vi "GUI main.vi"() -> ()   [LabVIEW 2020]
doc: "GUI of the control sotware. Entry VI that runs the whole control sotware."
uses:
  General DC meter/Type definitions/DC meter.ctl
  General DC meter/Type definitions/DC meter type.ctl
  General AC source/Type definitions/AC Source.ctl
  General AC source/Type definitions/AC Source type.ctl
  CE Measurement/Type definitions/CE measurement.ctl
  Utilities/Type definitions/Common properties.ctl
  FR Measurement/Type definitions/FR measuement.ctl
  General PJVS driver/Type definitions/PJVS.ctl
  General PJVS driver/Type definitions/PJVS Type.ctl
  external libraries/acsvcontrol-driver/Public/Type Definitions/Timeouts.ctl
  external libraries/JV modified NPL Bias source/DataSocketCluster external.ctl
  SS Measurement/Type definitions/SS measurement.ctl
  DG Measurement/DG measurement.ctl
  72cf5302-2c4c-4f5f-a6af-2a69e50c2212.vi
  <vilib>/Utility/error.llb/Error Cluster From Error Code.vi
  <vilib>/ErrorRing/Error Ring.xnode
  external libraries/varilib/varilib.lvlib
  external libraries/acsvcontrol-driver/ACSVcontrol-driver.lvlib
panel:
  out "DG measurement":T1={"Sampling frequencies (Hz)"=[10000000.0], "Requested PJVS frequencies (Hz)"=[1000.0], "Requested PJVS waveform amplitudes (V)"=[0.707], "Record lengths (multiples of PJVS periods)"=[10000.0], "Requested PJVS steps"=[20], "Switch position"=0.0, "Settle down after PJVS change (s)"=1.0, "Rs"=0, "Re"=0, "Algorithm"="TWM-PJVSSubS", "Calculate results"=FALSE, "Data folder"=path "", "TWM data directories"=[], "TWM data directories relative"=[], "DG measurement info files"=[], "Set PJVS frequencies (Hz)"=[1000.0], "Set PJVS reference voltages array of vector cluster"=[], "Set PJVS steps"=[1000]} {"Set PJVS frequencies (Hz)" format="%#_3p"; "Set PJVS reference voltages array of vector cluster"."PJVS reference voltages vector" format="%#_3p"; "Requested PJVS frequencies (Hz)" format="%#_3p"; "Record lengths (multiples of PJVS periods)" format="%#_3p"; "Sampling frequencies (Hz)" format="%#_3p"; "Requested PJVS waveform amplitudes (V)" format="%#_3p"}
  in  "DG setup":bool
  in  "DG measure":bool
  out "AC sync source":T2
  in  "DC manual":bool
  out "SS measurement":T4={"Signal frequencies (Hz)"=[1000.0], "Signal amplitudes (V)"=[0.707], "Sampling frequencies (Hz)"=[10000000.0], "Record lengths (multiples of periods)"=[10000.0], "Calculate results"=FALSE, "Algorithm"="TWM-WFFT", "TWM data directories"=[], "TWM data directories relative"=[], "Settle down after AC source change (s)"=1.0, "PJVS frequencies (Hz)"=[1000.0], "PJVS reference voltages array of vector cluster"=[{"PJVS reference voltages vector"=[]}], "Requested PJVS steps"=[20], "Measure CE"=FALSE, "Measure CE before"=FALSE, "Measure CE after"=FALSE, "Single point CE measurement"=FALSE, "original CE template path"=path "", "new CE template path before SS"=path "", "new CE template path before SS relative"=path "", "new CE template path after SS"=path "", "new CE template path after SS relative"=path "", "original CE fit path"=path "", "new CE fit path before SS"=path "", "new CE fit path before SS relative"=path "", "new CE fit path after SS"=path "", "new CE fit path after SS relative"=path "", "Measure digitizer gain"=FALSE, "Measure digitizer gain before"=FALSE, "Measure digitizer gain after"=FALSE, "Digitizer gain"=0.0, "Data folder"=path "", "FR fit path"=path "", "new FR fit path relative"=path "", "Rs"=0, "Re"=0, "SS measurement info files"=[]} {"PJVS reference voltages array of vector cluster"."PJVS reference voltages vector" format="%#_3p"; "PJVS frequencies (Hz)" format="%#_3p"; "Record lengths (multiples of periods)" format="%#_3p"; "Sampling frequencies (Hz)" format="%#_3p"; "Signal amplitudes (V)" format="%#_3p"; "Signal frequencies (Hz)" format="%#_3p"}
  out "PJVS":T5={"PJVS type"=enum."AC-supraVOLTcontrol", "Status Refnum"=refnum, "AC-supraVOLTcontrol"={"IP address:port (0.0.0.0:0000)"="0.0.0.0:0000", "Timeouts"={"TCP Read & Write (ms)"=7000, "Sensors readout"=5000, "PJVS setup"=10000, "Nullmeter readout"=5000, "Multiplexer setup"=3000, "57XX setup"=15000, "Generator setup"=5000, "Synthesizer setup"=3000, "Sampler readout"=10000}, "Simulation mode"=FALSE, "Debug mode"=FALSE}, "NPL bias source"={"DataSocketCluster"={"Server Machine"="CZC105BD8M", "Client Machine"="localhost", "Data"="P2", "TimeStamp"=0.0, "Count"=1, "Target Process"="General Server"}}, "Manual PJVS"={"PJVS frequency (Hz)"=0.0, "Reference voltages (V)"=[], "File with PJVS voltages"=path ""}, "VTT PJVS"={"some VTT only property"=""}} {"NPL bias source"."DataSocketCluster"."TimeStamp" format="%.2f"}
  out "FR measurement":T9={"Measurement frequencies (Hz)"=[1000.0, 10000.0, 1000.0], "Sampling frequency (Hz)"=500000.0, "Signal amplitude (V)"=4.5, "AC-DC settle time (s)"=20.0, "Record length (multiples of period)"=[1000.0, 10000.0, 1000.0], "Measurement template file"=path "", "Row of START keyword"=0, "Row of STOP keyword"=0, "Calculate RMS from samples"=FALSE, "AC-DC warm up time (s)"=300.0, "Measurement template line"=[], "DC meter readings No."=10, "Algorithm"="TWM-WFFT", "Simultaneous measurement"=FALSE, "Recalculate-skip already calculated"=FALSE} {"Record length (multiples of period)" format="%#_3p"; "Sampling frequency (Hz)" format="%#_3p"; "Measurement frequencies (Hz)" format="%#_3p"}
  in  "DS setup":bool
  in  "DS measure":bool
  in  "SS setup":bool
  in  "SS measure":bool
  out "Common properties":T10={"Measurement status ref"=refnum, "TWM Status ref"=refnum, "Abort ref"=refnum, "Skip waiting ref"=refnum, "GNU Octave path"=path "C:/Program Files/GNU Octave/Octave-6.2.0/mingw64/bin", "TWM+QWTB path"=path "C:/Users/labina/Desktop/TWM-1.8.7.0-full/octprog", "lvlib path"=path "D:/martin/WAC/WACsw - github/control_software/Filter function meter/external libraries/GOLPI 0.7.3.1 source distribution LV 20.0 32 bit/lv_proc.dll", "TWM pipe"="\\\\.\\pipe\\TWM:server", "PJVS status ref"=refnum, "WAC path"=path ""}
  out "CE measurement":T11={"Signal frequencies (Hz) T"=[1000.0], "Signal amplitudes (V) T"=[0.707], "Sampling frequencies (Hz) T"=[10000000.0], "Record lengths (multiples of periods) T"=[10000.0], "TWM data root directory"=path "", "TWM mreasurements directories"=[], "Calculate RMS from samples"=FALSE, "Algorithm to use"="TWM-WFFT", "Quantity to read"="TWM-WFFT", "Settle down after AC source change (s) T"=1.0, "Skip PJVS setup"=FALSE, "Measurement template file"=path "", "Row of START keyword T"=0, "Row of STOP keyword T"=0, "Measurement template line T"=[], "Switch position T"=[10000.0], "FR fit mat file T"=path "", "Recalculate-skip already calculated"=FALSE} {"Switch position T" format="%#_3p"; "Record lengths (multiples of periods) T" format="%#_3p"; "Sampling frequencies (Hz) T" format="%#_3p"; "Signal amplitudes (V) T" format="%#_3p"; "Signal frequencies (Hz) T" format="%#_3p"}
  in  "CE setup":bool
  in  "CE measure":bool
  out "AC Source":T2
  out "DC meter":T12={"DC meter type"=enum."H/A/K 3458", "DC meter VISA"="", "NPLC"=10.0, "status ref"=refnum}
  in  "PJVS setup":bool
  out "PJVS status":string caption="PJVS:"
  out "gui_to_hide":refnum<vi>[](array[refnum])
  in  "Skip waiting":bool caption="Abort"
  in  "DCV setup":bool
  out "DC meter status":string caption="DC meter:"
  out "Measurement status:":string
  in  "AC setup":bool
  in  "FR measure":bool
  out "gui_unlock_for_measure":refnum<vi>[](array[refnum])
  out "gui_to_lock":refnum<vi>[](array[refnum])
  in  "FR setup":bool
  in  "Abort":bool
  out "AC source status":string caption="AC source:"
  out "TWM status":string caption="TWM:"
  in  "TWM setup":bool
  in  "About":bool
  in  "Quit":bool
  in  "ACmanual":bool
  in  "PJVSmanual":bool
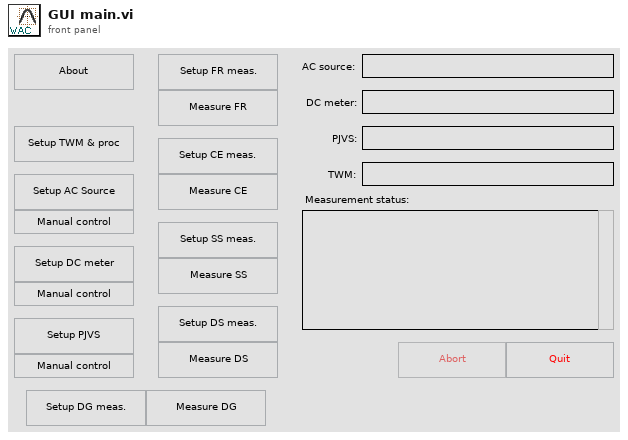
[diagram p1: front panel]
types:
  T1 = typedef "DG measurement.ctl" = cluster{"Sampling frequencies (Hz)":dbl[], "Requested PJVS frequencies (Hz)":dbl[], "Requested PJVS waveform amplitudes (V)":dbl[], "Record lengths (multiples of PJVS periods)":dbl[], "Requested PJVS steps":u32[], "Switch position":dbl, "Settle down after PJVS change (s)":dbl, "Rs":i32, "Re":i32, "Algorithm":string, "Calculate results":bool, "Data folder":path, "TWM data directories":path[], "TWM data directories relative":path[], "DG measurement info files":path[], "Set PJVS frequencies (Hz)":dbl[], "Set PJVS reference voltages array of vector cluster":cluster{"PJVS reference voltages vector":dbl[]}[], "Set PJVS steps":u32[]}
  T2 = typedef "AC Source.ctl" = cluster{"AC Source type":T3, "VISA":refnum<visa-resource-name>, "Ref. clock (Hz)":dbl, "status ref":refnum<vi>, "Fluke 57XX wideband output":bool, "Fluke 57XX ignore errors":bool, "Synchronization by AC signal":bool}
  T3 = typedef "AC Source type.ctl" = enum16{"Fluke 5XXX calibrator", "Tektronix AFG3000 series", "dummy", "Agilent 331xxA to 332xxA", "Agilent 335xxA to 336xxA"}
  T4 = typedef "SS measurement.ctl" = cluster{"Signal frequencies (Hz)":dbl[], "Signal amplitudes (V)":dbl[], "Sampling frequencies (Hz)":dbl[], "Record lengths (multiples of periods)":dbl[], "Calculate results":bool, "Algorithm":string, "TWM data directories":path[], "TWM data directories relative":path[], "Settle down after AC source change (s)":dbl, "PJVS frequencies (Hz)":dbl[], "PJVS reference voltages array of vector cluster":cluster{"PJVS reference voltages vector":dbl[]}[], "Requested PJVS steps":u32[], "Measure CE":bool, "Measure CE before":bool, "Measure CE after":bool, "Single point CE measurement":bool, "original CE template path":path, "new CE template path before SS":path, "new CE template path before SS relative":path, "new CE template path after SS":path, "new CE template path after SS relative":path, "original CE fit path":path, "new CE fit path before SS":path, "new CE fit path before SS relative":path, "new CE fit path after SS":path, "new CE fit path after SS relative":path, "Measure digitizer gain":bool, "Measure digitizer gain before":bool, "Measure digitizer gain after":bool, "Digitizer gain":dbl, "Data folder":path, "FR fit path":path, "new FR fit path relative":path, "Rs":i32, "Re":i32, "SS measurement info files":path[]}
  T5 = typedef "PJVS.ctl" = cluster{"PJVS type":T6, "Status Refnum":refnum<vi>, "AC-supraVOLTcontrol":cluster{"IP address:port (0.0.0.0:0000)":string, "Timeouts":T7, "Simulation mode":bool, "Debug mode":bool}, "NPL bias source":cluster{"DataSocketCluster":T8}, "Manual PJVS":cluster{"PJVS frequency (Hz)":dbl, "Reference voltages (V)":dbl[], "File with PJVS voltages":path}, "VTT PJVS":cluster{"some VTT only property":string}}
  T6 = typedef "PJVS Type.ctl" = enum16{"AC-supraVOLTcontrol", "JV modified NPL bias control", "Manual PJVS", "VTT PJVS"}
  T7 = typedef "ACSVcontrol-driver.lvlib/Timeouts.ctl" = cluster{"TCP Read & Write (ms)":i32, "Sensors readout":i32, "PJVS setup":i32, "Nullmeter readout":i32, "Multiplexer setup":i32, "57XX setup":i32, "Generator setup":i32, "Synthesizer setup":i32, "Sampler readout":i32}
  T8 = typedef "DataSocketCluster external.ctl" = cluster{"Server Machine":string, "Client Machine":string, "Data":string, "TimeStamp":dbl, "Count":i32, "Target Process":string}
  T9 = typedef "FR measuement.ctl" = cluster{"Measurement frequencies (Hz)":dbl[], "Sampling frequency (Hz)":dbl, "Signal amplitude (V)":dbl, "AC-DC settle time (s)":dbl, "Record length (multiples of period)":dbl[], "Measurement template file":path, "Row of START keyword":i32, "Row of STOP keyword":i32, "Calculate RMS from samples":bool, "AC-DC warm up time (s)":dbl, "Measurement template line":i32[], "DC meter readings No.":i32, "Algorithm":string, "Simultaneous measurement":bool, "Recalculate-skip already calculated":bool}
  T10 = typedef "Common properties.ctl" = cluster{"Measurement status ref":refnum<vi>, "TWM Status ref":refnum<vi>, "Abort ref":refnum<vi>, "Skip waiting ref":refnum<vi>, "GNU Octave path":path, "TWM+QWTB path":path, "lvlib path":path, "TWM pipe":string, "PJVS status ref":refnum<vi>, "WAC path":path}
  T11 = typedef "CE measurement.ctl" = cluster{"Signal frequencies (Hz) T":dbl[], "Signal amplitudes (V) T":dbl[], "Sampling frequencies (Hz) T":dbl[], "Record lengths (multiples of periods) T":dbl[], "TWM data root directory":path, "TWM mreasurements directories":path[], "Calculate RMS from samples":bool, "Algorithm to use":string, "Quantity to read":string, "Settle down after AC source change (s) T":dbl, "Skip PJVS setup":bool, "Measurement template file":path, "Row of START keyword T":i32, "Row of STOP keyword T":i32, "Measurement template line T":i32[], "Switch position T":dbl[], "FR fit mat file T":path, "Recalculate-skip already calculated":bool}
  T12 = typedef "DC meter.ctl" = cluster{"DC meter type":T13, "DC meter VISA":refnum<visa-resource-name>, "NPLC":dbl, "status ref":refnum<vi>}
  T13 = typedef "DC meter type.ctl" = enum16{"H/A/K 3458", "Fluke 8508A", "dummy", "Keithley 2182"}
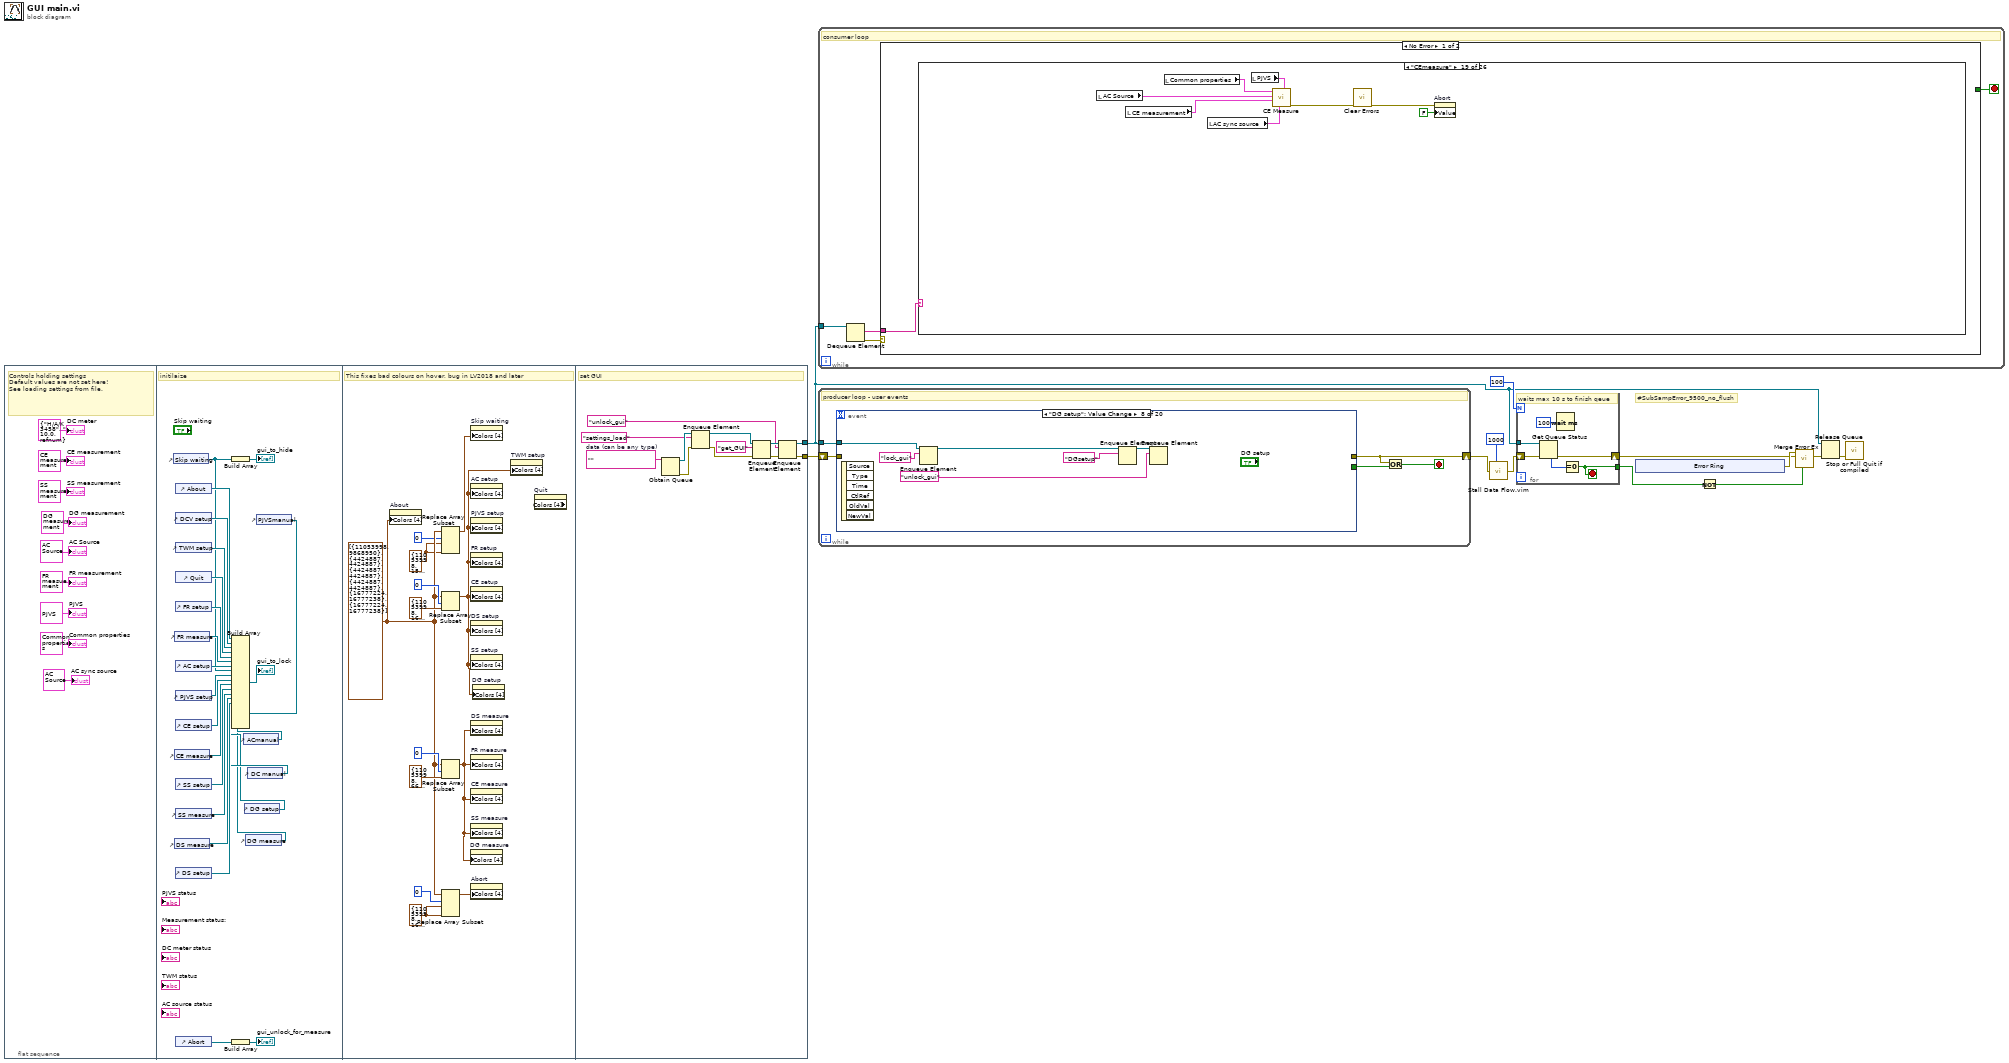
[diagram p0: block diagram]
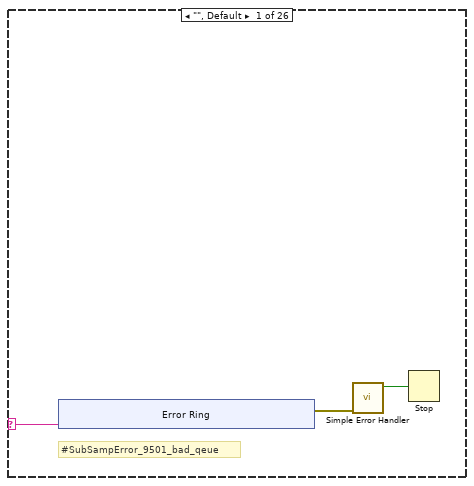
[diagram p2: hidden frame]
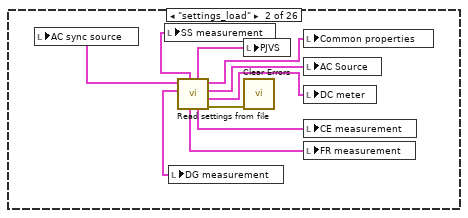
[diagram p3: hidden frame]
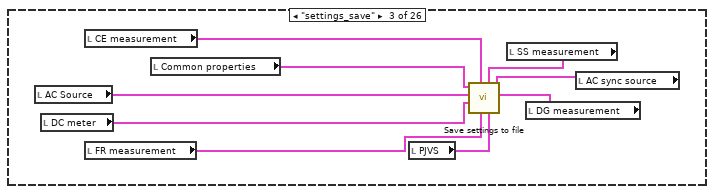
[diagram p4: hidden frame]
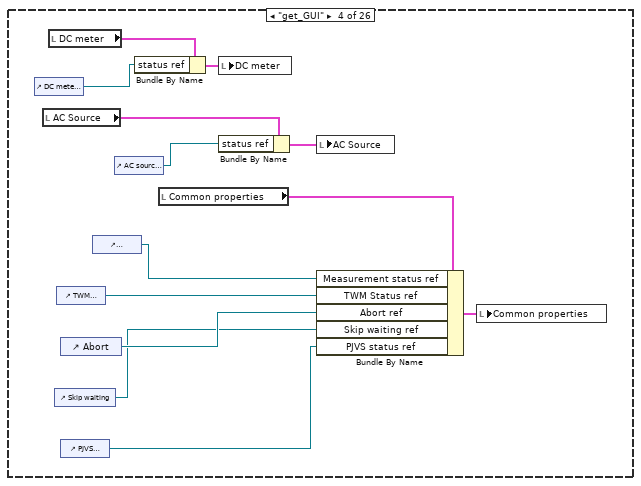
[diagram p5: hidden frame]
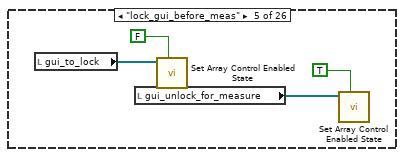
[diagram p6: hidden frame]
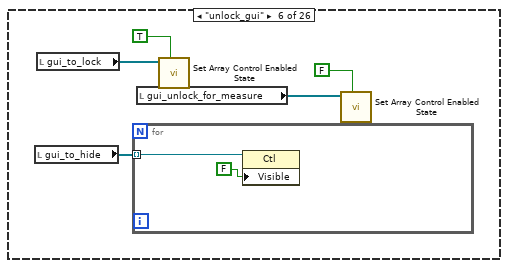
[diagram p7: hidden frame]
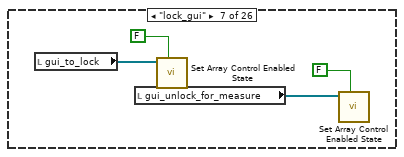
[diagram p8: hidden frame]
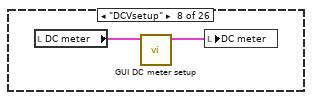
[diagram p9: hidden frame]
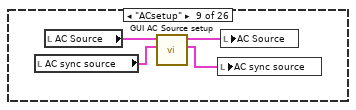
[diagram p10: hidden frame]
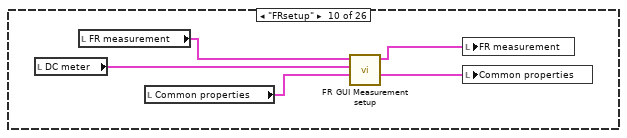
[diagram p11: hidden frame]
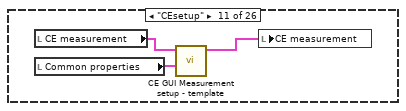
[diagram p12: hidden frame]
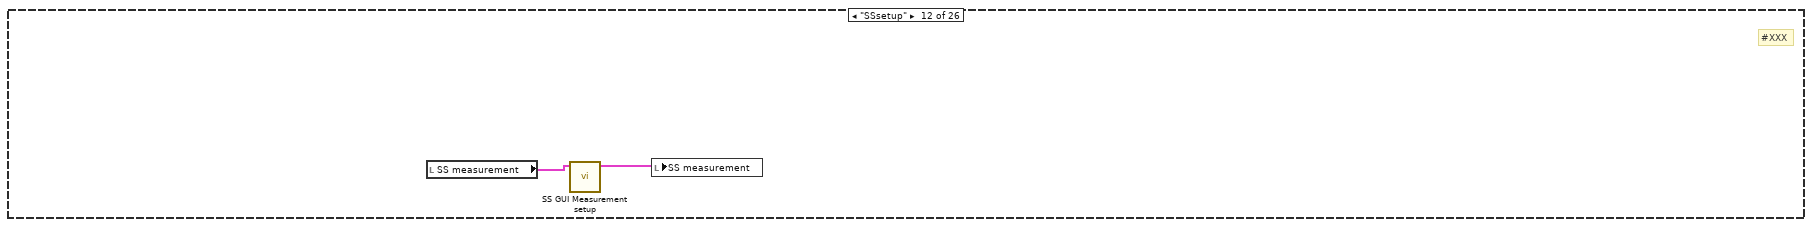
[diagram p13: hidden frame]
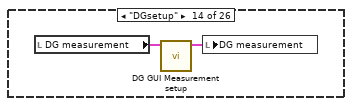
[diagram p15: hidden frame]
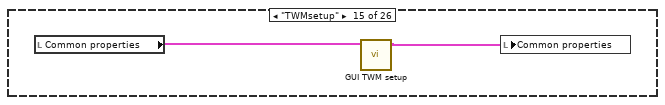
[diagram p16: hidden frame]
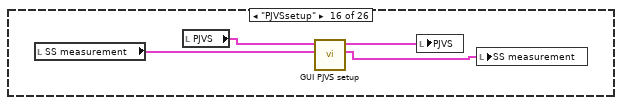
[diagram p17: hidden frame]
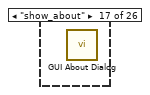
[diagram p18: hidden frame]
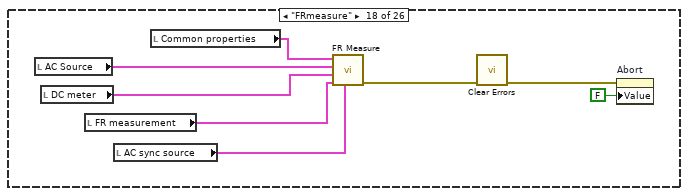
[diagram p19: hidden frame]
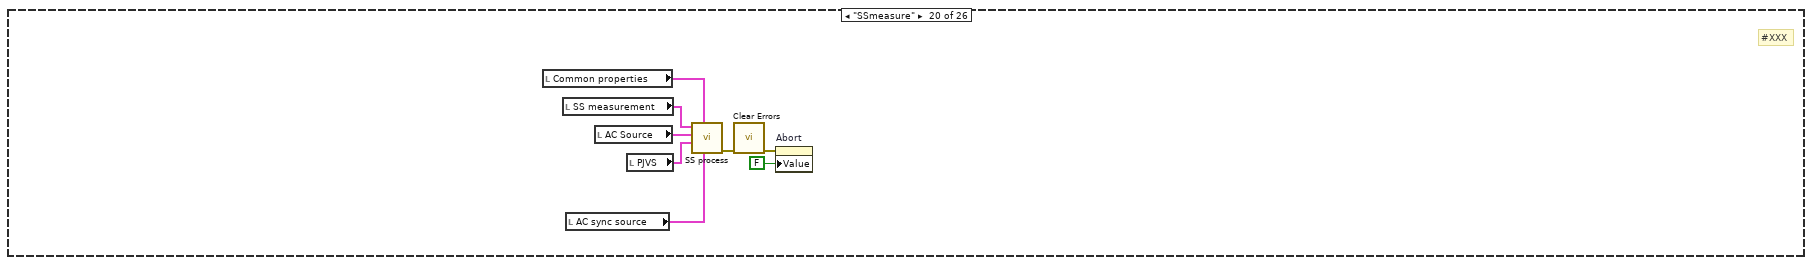
[diagram p20: hidden frame]
diagram:
  # "#SubSampError_9500_no_flush"
  n1 = flat-sequence {
    tunnel: [w65] -> w6
    tunnel: [w62] -> w12
    frame #0 {
      # "Controls holding settings\nDefault values are not set here!\nSee loading settings from file."
      "DC meter" <- T12 {"DC meter type"=enum."H/A/K 3458", "DC meter VISA"="", "NPLC"=10.0, "status ref"=refnum} ("DC meter")
      "AC Source" <- T2 {"AC Source type"=enum."Fluke 5XXX calibrator", "VISA"="", "Ref. clock (Hz)"=0.0, "status ref"=refnum, "Fluke 57XX wideband output"=FALSE, "Fluke 57XX ignore errors"=FALSE, "Synchronization by AC signal"=FALSE} ("AC Source")
      "Common properties" <- T10 {"Measurement status ref"=refnum, "TWM Status ref"=refnum, "Abort ref"=refnum, "Skip waiting ref"=refnum, "GNU Octave path"=path "C:/Program Files/GNU Octave/Octave-6.2.0/mingw64/bin", "TWM+QWTB path"=path "C:/Users/labina/Desktop/TWM-1.8.7.0-full/octprog", "lvlib path"=path "D:/martin/WAC/WACsw - github/control_software/Filter function meter/external libraries/GOLPI 0.7.3.1 source distribution LV 20.0 32 bit/lv_proc.dll", "TWM pipe"="\\\\.\\pipe\\TWM:server", "PJVS status ref"=refnum, "WAC path"=path ""} ("Common properties")
      "CE measurement" <- T11 {"Signal frequencies (Hz) T"=[1000.0], "Signal amplitudes (V) T"=[0.707], "Sampling frequencies (Hz) T"=[10000000.0], "Record lengths (multiples of periods) T"=[10000.0], "TWM data root directory"=path "", "TWM mreasurements directories"=[], "Calculate RMS from samples"=FALSE, "Algorithm to use"="TWM-WFFT", "Quantity to read"="TWM-WFFT", "Settle down after AC source change (s) T"=1.0, "Skip PJVS setup"=FALSE, "Measurement template file"=path "", "Row of START keyword T"=0, "Row of STOP keyword T"=0, "Measurement template line T"=[], "Switch position T"=[10000.0], "FR fit mat file T"=path "", "Recalculate-skip already calculated"=FALSE} ("CE measurement properties")
      "FR measurement" <- T9 {"Measurement frequencies (Hz)"=[1000.0, 10000.0, 1000.0], "Sampling frequency (Hz)"=500000.0, "Signal amplitude (V)"=4.5, "AC-DC settle time (s)"=20.0, "Record length (multiples of period)"=[1000.0, 10000.0, 1000.0], "Measurement template file"=path "", "Row of START keyword"=0, "Row of STOP keyword"=0, "Calculate RMS from samples"=FALSE, "AC-DC warm up time (s)"=300.0, "Measurement template line"=[], "DC meter readings No."=10, "Algorithm"="TWM-WFFT", "Simultaneous measurement"=FALSE, "Recalculate-skip already calculated"=FALSE} ("FR measurement")
      "PJVS" <- T5 {"PJVS type"=enum."AC-supraVOLTcontrol", "Status Refnum"=refnum, "AC-supraVOLTcontrol"={"IP address:port (0.0.0.0:0000)"="0.0.0.0:0000", "Timeouts"={"TCP Read & Write (ms)"=7000, "Sensors readout"=5000, "PJVS setup"=10000, "Nullmeter readout"=5000, "Multiplexer setup"=3000, "57XX setup"=15000, "Generator setup"=5000, "Synthesizer setup"=3000, "Sampler readout"=10000}, "Simulation mode"=FALSE, "Debug mode"=FALSE}, "NPL bias source"={"DataSocketCluster"={"Server Machine"="CZC105BD8M", "Client Machine"="localhost", "Data"="P2", "TimeStamp"=0.0, "Count"=1, "Target Process"="General Server"}}, "Manual PJVS"={"PJVS frequency (Hz)"=0.0, "Reference voltages (V)"=[], "File with PJVS voltages"=path ""}, "VTT PJVS"={"some VTT only property"=""}} ("PJVS")
      "SS measurement" <- T4 {"Signal frequencies (Hz)"=[1000.0], "Signal amplitudes (V)"=[0.707], "Sampling frequencies (Hz)"=[10000000.0], "Record lengths (multiples of periods)"=[10000.0], "Calculate results"=FALSE, "Algorithm"="TWM-WFFT", "TWM data directories"=[], "TWM data directories relative"=[], "Settle down after AC source change (s)"=1.0, "PJVS frequencies (Hz)"=[1000.0], "PJVS reference voltages array of vector cluster"=[{"PJVS reference voltages vector"=[]}], "Requested PJVS steps"=[20], "Measure CE"=FALSE, "Measure CE before"=FALSE, "Measure CE after"=FALSE, "Single point CE measurement"=FALSE, "original CE template path"=path "", "new CE template path before SS"=path "", "new CE template path before SS relative"=path "", "new CE template path after SS"=path "", "new CE template path after SS relative"=path "", "original CE fit path"=path "", "new CE fit path before SS"=path "", "new CE fit path before SS relative"=path "", "new CE fit path after SS"=path "", "new CE fit path after SS relative"=path "", "Measure digitizer gain"=FALSE, "Measure digitizer gain before"=FALSE, "Measure digitizer gain after"=FALSE, "Digitizer gain"=0.0, "Data folder"=path "", "FR fit path"=path "", "new FR fit path relative"=path "", "Rs"=0, "Re"=0, "SS measurement info files"=[]} ("SS measurement")
      "AC sync source" <- T2 {"AC Source type"=enum."Fluke 5XXX calibrator", "VISA"="", "Ref. clock (Hz)"=0.0, "status ref"=refnum, "Fluke 57XX wideband output"=FALSE, "Fluke 57XX ignore errors"=FALSE, "Synchronization by AC signal"=FALSE} ("AC Source")
      "DG measurement" <- T1 {"Sampling frequencies (Hz)"=[10000000.0], "Requested PJVS frequencies (Hz)"=[1000.0], "Requested PJVS waveform amplitudes (V)"=[0.707], "Record lengths (multiples of PJVS periods)"=[10000.0], "Requested PJVS steps"=[20], "Switch position"=0.0, "Settle down after PJVS change (s)"=1.0, "Rs"=0, "Re"=0, "Algorithm"="TWM-PJVSSubS", "Calculate results"=FALSE, "Data folder"=path "", "TWM data directories"=[], "TWM data directories relative"=[], "DG measurement info files"=[], "Set PJVS frequencies (Hz)"=[1000.0], "Set PJVS reference voltages array of vector cluster"=[], "Set PJVS steps"=[1000]} ("DG measurement")
    }
    frame #1 {
      # "initilaize"
      n2 = control-ref of="Skip waiting"() -> (w35:refnum<vi>)
      n3 = control-ref of="FR measure"() -> (w38:refnum<vi>)
      n4 = control-ref of="CE measure"() -> (w31:refnum<vi>)
      n5 = control-ref of="DS measure"() -> (w28:refnum<vi>)
      n6 = control-ref of="About"() -> (w39:refnum<vi>)
      n7 = control-ref of="DCV setup"() -> (w36:refnum<vi>)
      n8 = control-ref of="TWM setup"() -> (w40:refnum<vi>)
      n9 = control-ref of="Quit"() -> (w41:refnum<vi>)
      n10 = control-ref of="FR setup"() -> (w42:refnum<vi>)
      n11 = control-ref of="AC setup"() -> (w37:refnum<vi>)
      n12 = control-ref of="PJVS setup"() -> (w33:refnum<vi>)
      n13 = control-ref of="CE setup"() -> (w32:refnum<vi>)
      n14 = control-ref of="SS setup"() -> (w30:refnum<vi>)
      n15 = control-ref of="SS measure"() -> (w29:refnum<vi>)
      n16 = control-ref of="DS setup"() -> (w27:refnum<vi>)
      n17 = control-ref of="Abort"() -> (w43:refnum<vi>)
      n18 = Build Array(w35) -> (→"gui_to_hide":refnum<vi>[])
      n19 = Build Array(w43) -> (→"gui_unlock_for_measure":refnum<vi>[])
      n20 = control-ref of="ACmanual"() -> (w25:refnum<vi>)
      n21 = control-ref of="DG setup"() -> (w23:refnum<vi>)
      n22 = control-ref of="DG measure"() -> (w22:refnum<vi>)
      n23 = control-ref of="DC manual"() -> (w24:refnum<vi>)
      n24 = control-ref of="PJVSmanual"() -> (w26:refnum<vi>)
      n25 = Build Array(w39, w36, w40, w41, w42, w38, w37, w35, w33, w32, w31, w30, w29, w28, w27, w26, w25, w24, w23, w22) -> (→"gui_to_lock":refnum<vi>[])
    }
    frame #2 {
      w49 = cluster{u32, u32} {11053998, 15466424}
      w48 = cluster{u32, u32} {11053998, 16748945}
      w52 = cluster{u32, u32}[] [{11053998, 9868950}, {4424887, 4424887}, {4424887, 4424887}, {4424887, 4424887}, {16777224, 16777238}, {16777224, 16777238}] ("Colors [4]")
      # "This fixes bad colours on hover, bug in LV2018 and later"
      n26 = property on="About" class="Bool"("Colors [4]"=w52) -> ()  [unwired: 2 in, 2 out]
      n27 = Replace Array Subset(array=w52, new element #1=w49, index #1=0 ("index"), new element #2=w49) -> (w51:cluster{u32, u32}[])  [unwired: 1 in]
      n28 = Replace Array Subset(array=w52, new element=cluster{u32, u32} {11053998, 16776960}, index=0) -> (w47:cluster{u32, u32}[])
      n29 = Replace Array Subset(array=w52, new element=cluster{u32, u32} {11053998, 6618880}, index=0) -> (w46:cluster{u32, u32}[])
      n30 = Replace Array Subset(array=w52, new element #1=w48, index #1=0 ("index"), new element #2=w48) -> (w58:cluster{u32, u32}[])  [unwired: 1 in]
      n31 = property on="DG measure" class="Bool"("Colors [4]"=w46) -> ()  [unwired: 2 in, 2 out]
      n32 = property on="Skip waiting" class="Bool (strict)"("Colors [4]"=w51) -> ()  [unwired: 2 in, 2 out]
      n33 = property on="AC setup" class="Bool"("Colors [4]"=w47) -> ()  [unwired: 2 in, 2 out]
      n34 = property on="PJVS setup" class="Bool"("Colors [4]"=w47) -> ()  [unwired: 2 in, 2 out]
      n35 = property on="FR setup" class="Bool"("Colors [4]"=w47) -> ()  [unwired: 2 in, 2 out]
      n36 = property on="CE setup" class="Bool"("Colors [4]"=w47) -> ()  [unwired: 2 in, 2 out]
      n37 = property on="DS setup" class="Bool"("Colors [4]"=w47) -> ()  [unwired: 2 in, 2 out]
      n38 = property on="SS setup" class="Bool"("Colors [4]"=w47) -> ()  [unwired: 2 in, 2 out]
      n39 = property on="DS measure" class="Bool"("Colors [4]"=w46) -> ()  [unwired: 2 in, 2 out]
      n40 = property on="FR measure" class="Bool"("Colors [4]"=w46) -> ()  [unwired: 2 in, 2 out]
      n41 = property on="CE measure" class="Bool"("Colors [4]"=w46) -> ()  [unwired: 2 in, 2 out]
      n42 = property on="SS measure" class="Bool"("Colors [4]"=w46) -> ()  [unwired: 2 in, 2 out]
      n43 = property on="Abort" class="Bool (strict)"("Colors [4]"=w58) -> ()  [unwired: 2 in, 2 out]
      n44 = property on="DG setup" class="Bool"("Colors [4]"=w47) -> ()  [unwired: 2 in, 2 out]
      n45 = property on="TWM setup" class="Bool"("Colors [4]"=w47) -> ()  [unwired: 2 in, 2 out]
      n46 = property on="Quit" class="Bool" props=["Colors [4]"]() -> ()  [unwired: 2 in, 3 out]
    }
    frame #3 {
      w70 = ""  # data (can be any type)
      # "set GUI"
      n47 = Obtain Queue(element data type=w70) -> (queue out=w69:refnum<queue>, error out=w68:errorcluster)  [unwired: 4 in, 1 out]
      n48 = Enqueue Element(queue=w69, element="settings_load", error in (no error)=w68) -> (queue out=w60:refnum<queue>, error out=w59:errorcluster)  [unwired: 1 in, 1 out]
      n49 = Enqueue Element(queue=w60, element="get_GUI", error in (no error)=w59) -> (queue out=w63:refnum<queue>, error out=w64:errorcluster)  [unwired: 1 in, 1 out]
      n50 = Enqueue Element(queue=w63, element="unlock_gui", error in (no error)=w64) -> (queue out=w65:refnum<queue>, error out=w62:errorcluster)  [unwired: 1 in, 1 out]
    }
  }
  n51 = while {
    tunnel: w6 -> [w74]
    stop <- w71 stop-if-true
    # "consumer loop"
    n52 = Dequeue Element(queue=w74) -> (element=w72:string, error out=w73:errorcluster)  [unwired: 2 in, 2 out]
    n53 = case shown="No Error" w73 {
      tunnel: w72 -> [w75 _]
      tunnel: [_ TRUE] -> w71
      frame No Error {
        n54 = case shown="\"CEmeasure\"" w75 {
          selector: w75 -> [w76 _ _ _ _ _ _ _ _ _ _ _ _ _ _ _ _ _ _ _ _ _ _ _ _ _]
          frame "", Default {
            # "#SubSampError_9501_bad_qeue"
            n55 = xnode "Error Ring"("parameter 0"=w76) -> ("error out"=w78:errorcluster)
            n56 = call <vilib>:"Simple Error Handler.vi"("error in (no error)"=w78) -> ("error?"=w77:bool)  [unwired: 4 in, 4 out]
            n57 = Stop(stop? (T)=w77) -> ()
          }
          frame "settings_load" {
            n58 = call "Read settings from file.vi"() -> ("error out"=w95:errorcluster, "DC meter"=w92:T12, "AC Source"=w93:T2, "Common properties"=w94:T10, "CE measurement"=w91:T11, "PJVS"=w89:T5, "FR measurement"=w90:T9, "SS measurement"=w88:T4, "DG measurement"=w86:T1, "AC sync source"=w87:T2)  [unwired: 2 in]
            n59 = local write "AC sync source"(w87) -> ()
            n60 = local write "SS measurement"(w88) -> ()
            n61 = local write "DG measurement"(w86) -> ()
            n62 = local write "PJVS"(w89) -> ()
            n63 = call <vilib>:"Clear Errors.vi"("error in (no error)"=w95) -> ()  [unwired: 5 in, 2 out]
            n64 = local write "Common properties"(w94) -> ()
            n65 = local write "AC Source"(w93) -> ()
            n66 = local write "DC meter"(w92) -> ()
            n67 = local write "CE measurement"(w91) -> ()
            n68 = local write "FR measurement"(w90) -> ()
          }
          frame "settings_save" {
            n69 = local read "AC Source"() -> (w103:T2)
            n70 = local read "DC meter"() -> (w102:T12)
            n71 = local read "CE measurement"() -> (w101:T11)
            n72 = local read "FR measurement"() -> (w100:T9)
            n73 = local read "Common properties"() -> (w104:T10)
            n74 = local read "PJVS"() -> (w99:T5)
            n75 = local read "SS measurement"() -> (w98:T4)
            n76 = local read "DG measurement"() -> (w96:T1)
            n77 = local read "AC sync source"() -> (w97:T2)
            n78 = call "Save settings to file.vi"("DG measurement"=w96, "AC sync source"=w97, "PJVS"=w99, "SS measurement"=w98, "FR measurement"=w100, "CE measurement properties"=w101, "DC meter"=w102, "AC Source"=w103, "Common properties"=w104) -> ()  [unwired: 2 in, 1 out]
          }
          frame "get_GUI" {
            n79 = control-ref of="DC meter status"() -> (w106:refnum<vi>)
            n80 = local read "AC Source"() -> (w111:T2)
            n81 = local read "DC meter"() -> (w107:T12)
            n82 = control-ref of="Skip waiting"() -> (w112:refnum<vi>)
            n83 = control-ref of="TWM status"() -> (w113:refnum<vi>)
            n84 = control-ref of="Abort"() -> (w115:refnum<vi>)
            n85 = control-ref of="PJVS status"() -> (w105:refnum<vi>)
            n86 = control-ref of="Measurement status:"() -> (w114:refnum<vi>)
            n87 = control-ref of="AC source status"() -> (w109:refnum<vi>)
            n88 = Bundle By Name(cluster=w107, "status ref"=w106) -> (w108:T12)
            n89 = local read "Common properties"() -> (w117:T10)
            n90 = local write "DC meter"(w108) -> ()
            n91 = Bundle By Name(cluster=w111, "status ref"=w109) -> (w110:T2)
            n92 = local write "AC Source"(w110) -> ()
            n93 = Bundle By Name(cluster=w117, "Measurement status ref"=w114, "TWM Status ref"=w113, "Abort ref"=w115, "Skip waiting ref"=w112, "PJVS status ref"=w105) -> (w116:T10)
            n94 = local write "Common properties"(w116) -> ()
          }
          frame "lock_gui_before_meas" {
            n95 = local read "gui_to_lock"() -> (w121:refnum<vi>[])
            n96 = local read "gui_unlock_for_measure"() -> (w119:refnum<vi>[])
            n97 = call "Set Array Control Enabled State.vi"("enabled (T)"=FALSE, "reference array in"=w121) -> ()  [unwired: 8 in, 2 out]
            n98 = call "Set Array Control Enabled State.vi"("enabled (T)"=TRUE, "reference array in"=w119) -> ()  [unwired: 8 in, 2 out]
          }
          frame "unlock_gui" {
            n99 = local read "gui_to_hide"() -> (w122:refnum<vi>[])
            n100 = local read "gui_to_lock"() -> (w126:refnum<vi>[])
            n101 = for {
              tunnel: w122 -> [w128] mode=indexing
              n102 = property class="Ctl"(reference=w128, "Visible"=FALSE) -> ()  [unwired: 1 in, 2 out]
            }
            n103 = local read "gui_unlock_for_measure"() -> (w125:refnum<vi>[])
            n104 = call "Set Array Control Enabled State.vi"("enabled (T)"=TRUE, "reference array in"=w126) -> ()  [unwired: 8 in, 2 out]
            n105 = call "Set Array Control Enabled State.vi"("enabled (T)"=FALSE, "reference array in"=w125) -> ()  [unwired: 8 in, 2 out]
          }
          frame "lock_gui" {
            n106 = local read "gui_to_lock"() -> (w132:refnum<vi>[])
            n107 = local read "gui_unlock_for_measure"() -> (w131:refnum<vi>[])
            n108 = call "Set Array Control Enabled State.vi"("enabled (T)"=FALSE, "reference array in"=w132) -> ()  [unwired: 8 in, 2 out]
            n109 = call "Set Array Control Enabled State.vi"("enabled (T)"=FALSE, "reference array in"=w131) -> ()  [unwired: 8 in, 2 out]
          }
          frame "DCVsetup" {
            n110 = local read "DC meter"() -> (w133:T12)
            n111 = call "GUI DC meter setup.vi"("DC meter"=w133) -> ("DC meter out"=w134:T12)  [unwired: 10 in]
            n112 = local write "DC meter"(w134) -> ()
          }
          frame "ACsetup" {
            n113 = local read "AC sync source"() -> (w136:T2)
            n114 = local read "AC Source"() -> (w137:T2)
            n115 = call "GUI AC Source setup.vi"("AC sync source"=w136, "AC Source"=w137) -> ("AC sync source out"=w135:T2, "AC Source out"=w138:T2)  [unwired: 8 in]
            n116 = local write "AC sync source"(w135) -> ()
            n117 = local write "AC Source"(w138) -> ()
          }
          frame "FRsetup" {
            n118 = local read "DC meter"() -> (w143:T12)
            n119 = local read "FR measurement"() -> (w140:T9)
            n120 = local read "Common properties"() -> (w142:T10)
            n121 = call "FR GUI Measurement setup.vi"("Common properties"=w142, "DC meter"=w143, "FR measurement"=w140) -> ("Common properties out"=w141:T10, "FR measurement out"=w139:T9)  [unwired: 5 in]
            n122 = local write "FR measurement"(w139) -> ()
            n123 = local write "Common properties"(w141) -> ()
          }
          frame "CEsetup" {
            n124 = local read "CE measurement"() -> (w146:T11)
            n125 = local read "Common properties"() -> (w144:T10)
            n126 = call "CE GUI Measurement setup - template.vi"("Common properties"=w144, "CE measurement"=w146) -> ("CE measurement out"=w145:T11)  [unwired: 7 in]
            n127 = local write "CE measurement"(w145) -> ()
          }
          frame "SSsetup" {
            # "#XXX"
            n128 = local read "SS measurement"() -> (w148:T4)
            n129 = call "SS GUI Measurement setup.vi"("SS measurement"=w148) -> ("SS measurement out"=w147:T4)  [unwired: 8 in]
            n130 = local write "SS measurement"(w147) -> ()
          }
          frame "DSsetup" {
            # "#XXX"
            # "#XXX"
          }
          frame "DGsetup" {
            n131 = local read "DG measurement"() -> (w150:T1)
            n132 = call "DG GUI Measurement setup.vi"("DG measurement"=w150) -> ("DG measurement out"=w149:T1)  [unwired: 8 in]
            n133 = local write "DG measurement"(w149) -> ()
          }
          frame "TWMsetup" {
            n134 = local read "Common properties"() -> (w152:T10)
            n135 = call "GUI TWM setup.vi"("Common properties"=w152) -> ("Common properties out"=w151:T10)  [unwired: 9 in]
            n136 = local write "Common properties"(w151) -> ()
          }
          frame "PJVSsetup" {
            n137 = local read "SS measurement"() -> (w155:T4)
            n138 = local read "PJVS"() -> (w156:T5)
            n139 = call "GUI PJVS setup.vi"("SS measurement"=w155, "PJVS"=w156) -> ("SS measurement out"=w153:T4, "PJVS out"=w154:T5)  [unwired: 8 in]
            n140 = local write "PJVS"(w154) -> ()
            n141 = local write "SS measurement"(w153) -> ()
          }
          frame "show_about" {
            n142 = call "GUI About Dialog.vi"() -> ()  [unwired: 12 in]
          }
          frame "FRmeasure" {
            n143 = local read "AC Source"() -> (w160:T2)
            n144 = local read "DC meter"() -> (w159:T12)
            n145 = local read "FR measurement"() -> (w158:T9)
            n146 = local read "AC sync source"() -> (w157:T2)
            n147 = local read "Common properties"() -> (w161:T10)
            n148 = call "FR Measure.vi"("AC sync source"=w157, "FR measurement"=w158, "DC meter"=w159, "AC Source"=w160, "Common properties"=w161) -> ("error out"=w164:errorcluster)  [unwired: 6 in]
            n149 = call <vilib>:"Clear Errors.vi"("error in (no error)"=w164) -> ("error out"=w163:errorcluster)  [unwired: 5 in, 1 out]
            n150 = property on="Abort" class="Bool (strict)"(error in=w163, "Value"=FALSE ("Abort")) -> ()  [unwired: 1 in, 2 out]
          }
          frame "CEmeasure" {
            n151 = local read "AC Source"() -> (w168:T2)
            n152 = local read "CE measurement"() -> (w167:T11)
            n153 = local read "Common properties"() -> (w169:T10)
            n154 = local read "AC sync source"() -> (w166:T2)
            n155 = local read "PJVS"() -> (w165:T5)
            n156 = call "CE Measure.vi"("PJVS setup"=w165, "AC sync source"=w166, "CE measurement"=w167, "AC Source"=w168, "Common properties"=w169) -> ("error out"=w170:errorcluster)  [unwired: 6 in]
            n157 = call <vilib>:"Clear Errors.vi"("error in (no error)"=w170) -> ("error out"=w172:errorcluster)  [unwired: 5 in, 1 out]
            n158 = property on="Abort" class="Bool (strict)"(error in=w172, "Value"=FALSE ("Abort")) -> ()  [unwired: 1 in, 2 out]
          }
          frame "SSmeasure" {
            # "#XXX"
            n159 = local read "Common properties"() -> (w179:T10)
            n160 = local read "SS measurement"() -> (w180:T4)
            n161 = local read "AC sync source"() -> (w173:T2)
            n162 = local read "AC Source"() -> (w178:T2)
            n163 = local read "PJVS"() -> (w177:T5)
            n164 = call "SS process.vi"("AC sync source"=w173, "Common properties"=w179, "PJVS"=w177, "AC Source"=w178, "SS measurement"=w180) -> ("error out"=w174:errorcluster)  [unwired: 6 in]
            n165 = call <vilib>:"Clear Errors.vi"("error in (no error)"=w174) -> ("error out"=w176:errorcluster)  [unwired: 5 in, 1 out]
            n166 = property on="Abort" class="Bool (strict)"(error in=w176, "Value"=FALSE ("Abort")) -> ()  [unwired: 1 in, 2 out]
          }
          frame "DSmeasure" {
            # "#XXX"
            # "#XXX"
          }
          frame "DGmeasure" {
            n167 = local read "Common properties"() -> (w184:T10)
            n168 = local read "DG measurement"() -> (w182:T1)
            n169 = local read "PJVS"() -> (w183:T5)
            n170 = call "DG Measure.vi"("PJVS setup"=w183, "DG measurement"=w182, "Common properties"=w184) -> ("error out"=w181:errorcluster)  [unwired: 8 in]
            n171 = call <vilib>:"Clear Errors.vi"("error in (no error)"=w181) -> ("error out"=w186:errorcluster)  [unwired: 5 in, 1 out]
            n172 = property on="Abort" class="Bool (strict)"(error in=w186, "Value"=FALSE ("Abort")) -> ()  [unwired: 1 in, 2 out]
          }
          frame "ACmanual" {
            n173 = vi-ref "AC Source manual control GUI.vi"() -> (w195:refnum<vi>)
            n174 = local read "AC Source"() -> (w192:T2)
            n175 = property class="VI"(reference=w195) -> (error out=w193:errorcluster, "Name"=w194:string)  [unwired: 1 in, 1 out]
            n176 = local read "AC sync source"() -> (w187:T2)
            n177 = Open VI Reference(type specifier VI Refnum (for type only)=refnum<vi> refnum, vi path=w194, options=128, error in (no error)=w193) -> (vi reference=w199:refnum<vi>, error out=w197:errorcluster)  [unwired: 2 in]
            n178 = call-by-ref "Start Asynchronous Call"(reference=w199, error in=w197, "AC sync source"=w187, "AC Source"=w192) -> (reference out=w191:refnum<vi>, error out=w190:errorcluster)  [unwired: 10 in]
            n179 = invoke class="VI (strict)" method="FP.Open"(reference=w191, error in=w190) -> (reference out=w188:refnum<vi>, error out=w189:errorcluster)  [unwired: 3 in, 3 out]
            n180 = Close Reference(reference=w188, error in (no error)=w189) -> ()  [unwired: 1 out]
          }
          frame "DCmanual" {
            n181 = vi-ref "DC meter manual control GUI.vi"() -> (w207:refnum<vi>)
            n182 = local read "DC meter"() -> (w204:T12)
            n183 = property class="VI"(reference=w207) -> (error out=w205:errorcluster, "Name"=w206:string)  [unwired: 1 in, 1 out]
            n184 = Open VI Reference(type specifier VI Refnum (for type only)=refnum<vi> refnum, vi path=w206, options=128, error in (no error)=w205) -> (vi reference=w211:refnum<vi>, error out=w209:errorcluster)  [unwired: 2 in]
            n185 = call-by-ref "Start Asynchronous Call"(reference=w211, error in=w209, "DC meter"=w204) -> (reference out=w203:refnum<vi>, error out=w202:errorcluster)  [unwired: 11 in]
            n186 = invoke class="VI (strict)" method="FP.Open"(reference=w203, error in=w202) -> (reference out=w200:refnum<vi>, error out=w201:errorcluster)  [unwired: 3 in, 3 out]
            n187 = Close Reference(reference=w200, error in (no error)=w201) -> ()  [unwired: 1 out]
          }
          frame "PJVSmanual" {
            n188 = vi-ref "PJVS manual control GUI.vi"() -> (w219:refnum<vi>)
            n189 = property class="VI"(reference=w219) -> (error out=w217:errorcluster, "Name"=w218:string)  [unwired: 1 in, 1 out]
            n190 = local read "PJVS"() -> (w216:T5)
            n191 = Open VI Reference(type specifier VI Refnum (for type only)=refnum<vi> refnum, vi path=w218, options=128, error in (no error)=w217) -> (vi reference=w223:refnum<vi>, error out=w221:errorcluster)  [unwired: 2 in]
            n192 = call-by-ref "Start Asynchronous Call"(reference=w223, error in=w221, "PJVS"=w216) -> (reference out=w215:refnum<vi>, error out=w212:errorcluster)  [unwired: 11 in]
            n193 = invoke class="VI (strict)" method="FP.Open"(reference=w215, error in=w212) -> (reference out=w214:refnum<vi>, error out=w213:errorcluster)  [unwired: 3 in, 3 out]
            n194 = Close Reference(reference=w214, error in (no error)=w213) -> ()  [unwired: 1 out]
          }
          frame "quit" {
            n195 = call "Stop Octave.vi"("Stop Octave? (T)"=TRUE) -> ("error out"=w224:errorcluster)  [unwired: 10 in]
            n196 = call <vilib>:"Clear Errors.vi"("error in (no error)"=w224) -> ()  [unwired: 5 in, 2 out]
          }
        }
      }
      frame Error {
        # "Return true in any case that should stop the loop."
      }
    }
  }
  n197 = while {
    shift-right: [w227] -> w3
    shift-left: w12 -> [w230]
    tunnel: w6 -> [w231]
    stop <- w228 stop-if-true
    # "producer loop - user events"
    n198 = event shown="[7] \"DG setup\": Value Change" {
      selector: _ -> [_ _ _ _ _ _ _ _ _ _ _ _ _ _ _ _ _ _ _ _]
      dyn-events: _ -> [_ _ _ _ _ _ _ _ _ _ _ _ _ _ _ _ _ _ _ _]
      timeout: _ -> [_ _ _ _ _ _ _ _ _ _ _ _ _ _ _ _ _ _ _ _]
      tunnel: w231 -> [w236 w241 w247 w253 w259 w265 w271 w275 w281 w285 w291 w300 w307 w314 w321 w324 w332 w336 w340 _]
      tunnel: w230 -> [_ _ _ _ _ _ _ _ _ _ _ _ _ _ _ _ w333 w335 w339 _]
      tunnel: [_ _ _ _ _ _ _ _ _ _ _ w295 w302 w309 w316 w323 w331 w334 w338 _] -> w227
      tunnel: [TRUE ("cancel") _ _ _ _ _ _ _ _ _ _ _ _ _ _ _ _ _ _ _] -> w229
      event "Quit": Value Change; Panel Close {
        # "Do it twice because we really want to wait\ntill octave ends and the \"finish qeue\" loop\nwould kill labview too early because the qeue\nwill get empty too soon."
        n199 = event-data() -> ()  [unwired: 1 in, 2 out]
        n200 = Enqueue Element(queue=w236, element="settings_save") -> (queue out=w234:refnum<queue>)  [unwired: 2 in, 2 out]
        n201 = Enqueue Element(queue=w234, element="quit") -> (queue out=w233:refnum<queue>)  [unwired: 2 in, 2 out]
        n202 = Enqueue Element(queue=w233, element="quit") -> ()  [unwired: 2 in, 3 out]
      }
      event "AC setup": Value Change {
        n203 = event-data() -> ()  [unwired: 1 in, 2 out]
        n204 = Enqueue Element(queue=w241, element="lock_gui") -> (queue out=w240:refnum<queue>)  [unwired: 2 in, 2 out]
        n205 = Enqueue Element(queue=w240, element="ACsetup") -> (queue out=w239:refnum<queue>)  [unwired: 2 in, 2 out]
        n206 = Enqueue Element(queue=w239, element="unlock_gui") -> ()  [unwired: 2 in, 3 out]
      }
      event "DCV setup": Value Change {
        n207 = event-data() -> ()  [unwired: 1 in, 2 out]
        n208 = Enqueue Element(queue=w247, element="lock_gui") -> (queue out=w246:refnum<queue>)  [unwired: 2 in, 2 out]
        n209 = Enqueue Element(queue=w246, element="DCVsetup") -> (queue out=w245:refnum<queue>)  [unwired: 2 in, 2 out]
        n210 = Enqueue Element(queue=w245, element="unlock_gui") -> ()  [unwired: 2 in, 3 out]
      }
      event "FR setup": Value Change {
        n211 = event-data() -> ()  [unwired: 1 in, 6 out]
        n212 = Enqueue Element(queue=w253, element="lock_gui") -> (queue out=w252:refnum<queue>)  [unwired: 2 in, 2 out]
        n213 = Enqueue Element(queue=w252, element="FRsetup") -> (queue out=w251:refnum<queue>)  [unwired: 2 in, 2 out]
        n214 = Enqueue Element(queue=w251, element="unlock_gui") -> ()  [unwired: 2 in, 3 out]
      }
      event "CE setup": Value Change {
        n215 = event-data() -> ()  [unwired: 1 in, 6 out]
        n216 = Enqueue Element(queue=w259, element="lock_gui") -> (queue out=w258:refnum<queue>)  [unwired: 2 in, 2 out]
        n217 = Enqueue Element(queue=w258, element="CEsetup") -> (queue out=w257:refnum<queue>)  [unwired: 2 in, 2 out]
        n218 = Enqueue Element(queue=w257, element="unlock_gui") -> ()  [unwired: 2 in, 3 out]
      }
      event "SS setup": Value Change {
        n219 = event-data() -> ()  [unwired: 1 in, 6 out]
        n220 = Enqueue Element(queue=w265, element="lock_gui") -> (queue out=w264:refnum<queue>)  [unwired: 2 in, 2 out]
        n221 = Enqueue Element(queue=w264, element="SSsetup") -> (queue out=w263:refnum<queue>)  [unwired: 2 in, 2 out]
        n222 = Enqueue Element(queue=w263, element="unlock_gui") -> ()  [unwired: 2 in, 3 out]
      }
      event "DS setup": Value Change {
        n223 = event-data() -> ()  [unwired: 1 in, 6 out]
        n224 = Enqueue Element(queue=w271, element="lock_gui") -> (queue out=w270:refnum<queue>)  [unwired: 2 in, 2 out]
        n225 = Enqueue Element(queue=w270, element="DSsetup") -> (queue out=w269:refnum<queue>)  [unwired: 2 in, 2 out]
        n226 = Enqueue Element(queue=w269, element="unlock_gui") -> ()  [unwired: 2 in, 3 out]
      }
      event "DG setup": Value Change {
        n227 = event-data() -> ()  [unwired: 1 in, 6 out]
        n228 = Enqueue Element(queue=w275, element="lock_gui") -> (queue out=w280:refnum<queue>)  [unwired: 2 in, 2 out]
        n229 = Enqueue Element(queue=w280, element="DGsetup") -> (queue out=w279:refnum<queue>)  [unwired: 2 in, 2 out]
        n230 = Enqueue Element(queue=w279, element="unlock_gui") -> ()  [unwired: 2 in, 3 out]
      }
      event "About": Value Change {
        n231 = event-data() -> ()  [unwired: 1 in, 2 out]
        n232 = Enqueue Element(queue=w281, element="show_about") -> ()  [unwired: 2 in, 3 out]
      }
      event "TWM setup": Value Change {
        n233 = event-data() -> ()  [unwired: 1 in, 2 out]
        n234 = Enqueue Element(queue=w285, element="lock_gui") -> (queue out=w284:refnum<queue>)  [unwired: 2 in, 2 out]
        n235 = Enqueue Element(queue=w284, element="TWMsetup") -> (queue out=w283:refnum<queue>)  [unwired: 2 in, 2 out]
        n236 = Enqueue Element(queue=w283, element="unlock_gui") -> ()  [unwired: 2 in, 3 out]
      }
      event "PJVS setup": Value Change {
        n237 = event-data() -> ()  [unwired: 1 in, 2 out]
        n238 = Enqueue Element(queue=w291, element="lock_gui") -> (queue out=w290:refnum<queue>)  [unwired: 2 in, 2 out]
        n239 = Enqueue Element(queue=w290, element="PJVSsetup") -> (queue out=w289:refnum<queue>)  [unwired: 2 in, 2 out]
        n240 = Enqueue Element(queue=w289, element="unlock_gui") -> ()  [unwired: 2 in, 3 out]
      }
      event "FR measure": Value Change {
        n241 = event-data() -> ()  [unwired: 1 in, 6 out]
        n242 = Enqueue Element(queue=w300, element="lock_gui_before_meas") -> (queue out=w299:refnum<queue>)  [unwired: 2 in, 2 out]
        n243 = Enqueue Element(queue=w299, element="FRmeasure") -> (queue out=w298:refnum<queue>)  [unwired: 2 in, 2 out]
        n244 = Enqueue Element(queue=w298, element="unlock_gui") -> (error out=w295:errorcluster)  [unwired: 2 in, 2 out]
      }
      event "CE measure": Value Change {
        n245 = event-data() -> ()  [unwired: 1 in, 6 out]
        n246 = Enqueue Element(queue=w307, element="lock_gui_before_meas") -> (queue out=w306:refnum<queue>)  [unwired: 2 in, 2 out]
        n247 = Enqueue Element(queue=w306, element="CEmeasure") -> (queue out=w305:refnum<queue>)  [unwired: 2 in, 2 out]
        n248 = Enqueue Element(queue=w305, element="unlock_gui") -> (error out=w302:errorcluster)  [unwired: 2 in, 2 out]
      }
      event "SS measure": Value Change {
        n249 = event-data() -> ()  [unwired: 1 in, 6 out]
        n250 = Enqueue Element(queue=w314, element="lock_gui_before_meas") -> (queue out=w313:refnum<queue>)  [unwired: 2 in, 2 out]
        n251 = Enqueue Element(queue=w313, element="SSmeasure") -> (queue out=w312:refnum<queue>)  [unwired: 2 in, 2 out]
        n252 = Enqueue Element(queue=w312, element="unlock_gui") -> (error out=w309:errorcluster)  [unwired: 2 in, 2 out]
      }
      event "DS measure": Value Change {
        n253 = event-data() -> ()  [unwired: 1 in, 6 out]
        n254 = Enqueue Element(queue=w321, element="lock_gui_before_meas") -> (queue out=w320:refnum<queue>)  [unwired: 2 in, 2 out]
        n255 = Enqueue Element(queue=w320, element="DSmeasure") -> (queue out=w319:refnum<queue>)  [unwired: 2 in, 2 out]
        n256 = Enqueue Element(queue=w319, element="unlock_gui") -> (error out=w316:errorcluster)  [unwired: 2 in, 2 out]
      }
      event "DG measure": Value Change {
        n257 = event-data() -> ()  [unwired: 1 in, 6 out]
        n258 = Enqueue Element(queue=w324, element="lock_gui_before_meas") -> (queue out=w329:refnum<queue>)  [unwired: 2 in, 2 out]
        n259 = Enqueue Element(queue=w329, element="DGmeasure") -> (queue out=w328:refnum<queue>)  [unwired: 2 in, 2 out]
        n260 = Enqueue Element(queue=w328, element="unlock_gui") -> (error out=w323:errorcluster)  [unwired: 2 in, 2 out]
      }
      event "ACmanual": Value Change {
        n261 = event-data() -> ()  [unwired: 1 in, 6 out]
        n262 = Enqueue Element(queue=w332, element="ACmanual", error in (no error)=w333) -> (error out=w331:errorcluster)  [unwired: 1 in, 2 out]
      }
      event "PJVSmanual": Value Change {
        n263 = event-data() -> ()  [unwired: 1 in, 6 out]
        n264 = Enqueue Element(queue=w336, element="PJVSmanual", error in (no error)=w335) -> (error out=w334:errorcluster)  [unwired: 1 in, 2 out]
      }
      event "DC manual": Value Change {
        n265 = event-data() -> ()  [unwired: 1 in, 6 out]
        n266 = Enqueue Element(queue=w340, element="DCmanual", error in (no error)=w339) -> (error out=w338:errorcluster)  [unwired: 1 in, 2 out]
      }
      event "Abort": Value Change {
        n267 = event-data() -> ()  [unwired: 1 in, 6 out]
        n268 = control-ref of="Abort"() -> (w343:refnum<vi>)
        n269 = call "Set Control Enabled State.vi"("enabled (T)"=FALSE, "reference in"=w343) -> ()  [unwired: 8 in, 2 out]
      }
    }
    n270 = Or(x=w227, y=w229) -> (x .or. y?=w228:bool)
  }
  n271 = call "Stall Data Flow.vim"("value in"=w3, "milliseconds to wait"=u32 1000) -> ("value out"=w2:errorcluster)  [unwired: 1 out]
  n272 = for {
    N: 100 -> [_]
    tunnel: w6 -> [w349]
    shift-right: [w347] -> w10
    shift-left: w2 -> [w348]
    tunnel: [w344] -> w8
    stop <- w344 stop-if-true
    # "waits max 10 s to finish qeue"
    n273 = Get Queue Status(queue=w349, error in (no error)=w348) -> (error out=w347:errorcluster, # elements in queue=w345:i32)  [unwired: 1 in, 6 out]
    n274 = Wait (ms)(milliseconds to wait=u32 100) -> ()  [unwired: 1 out]
    n275 = Equal To 0?(x=w345) -> (x = 0?=w344:bool)
  }
  n276 = xnode "Error Ring"() -> ("error out"=w11:errorcluster)
  n277 = Not(x=w8) -> (.not. x?=w9:bool)
  n278 = call "Merge Error Ex.vi"("Is error? (False)"=w9, "main error in (no error)"=w10, "second error in"=w11) -> ("error out"=w5:errorcluster)  [unwired: 8 in]
  n279 = Release Queue(queue=w6, error in (no error)=w5) -> (error out=w4:errorcluster)  [unwired: 1 in, 2 out]
  n280 = call "Stop or Full Quit if compiled.vi"("error in (no effect)"=w4) -> ()  [unwired: 3 in]
